vi "RenameVI.vi"(8 "error in (no error)":errorcluster, 11 "InitialName":string) -> (0 "error out":errorcluster, 3 "NewName":string)   [LabVIEW 2018]
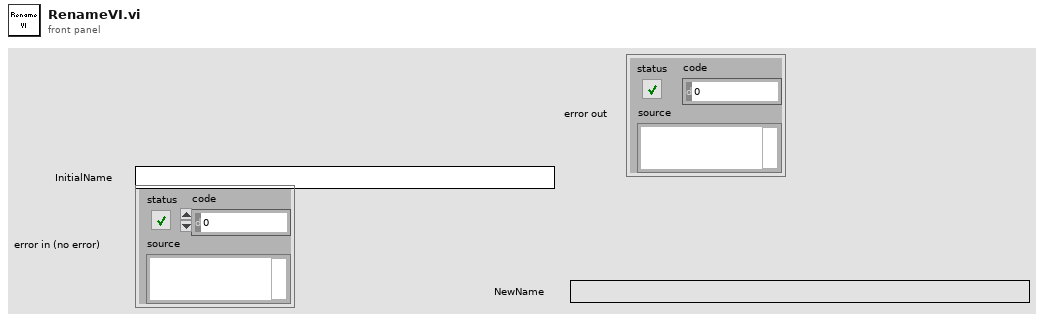
[diagram p1: front panel]
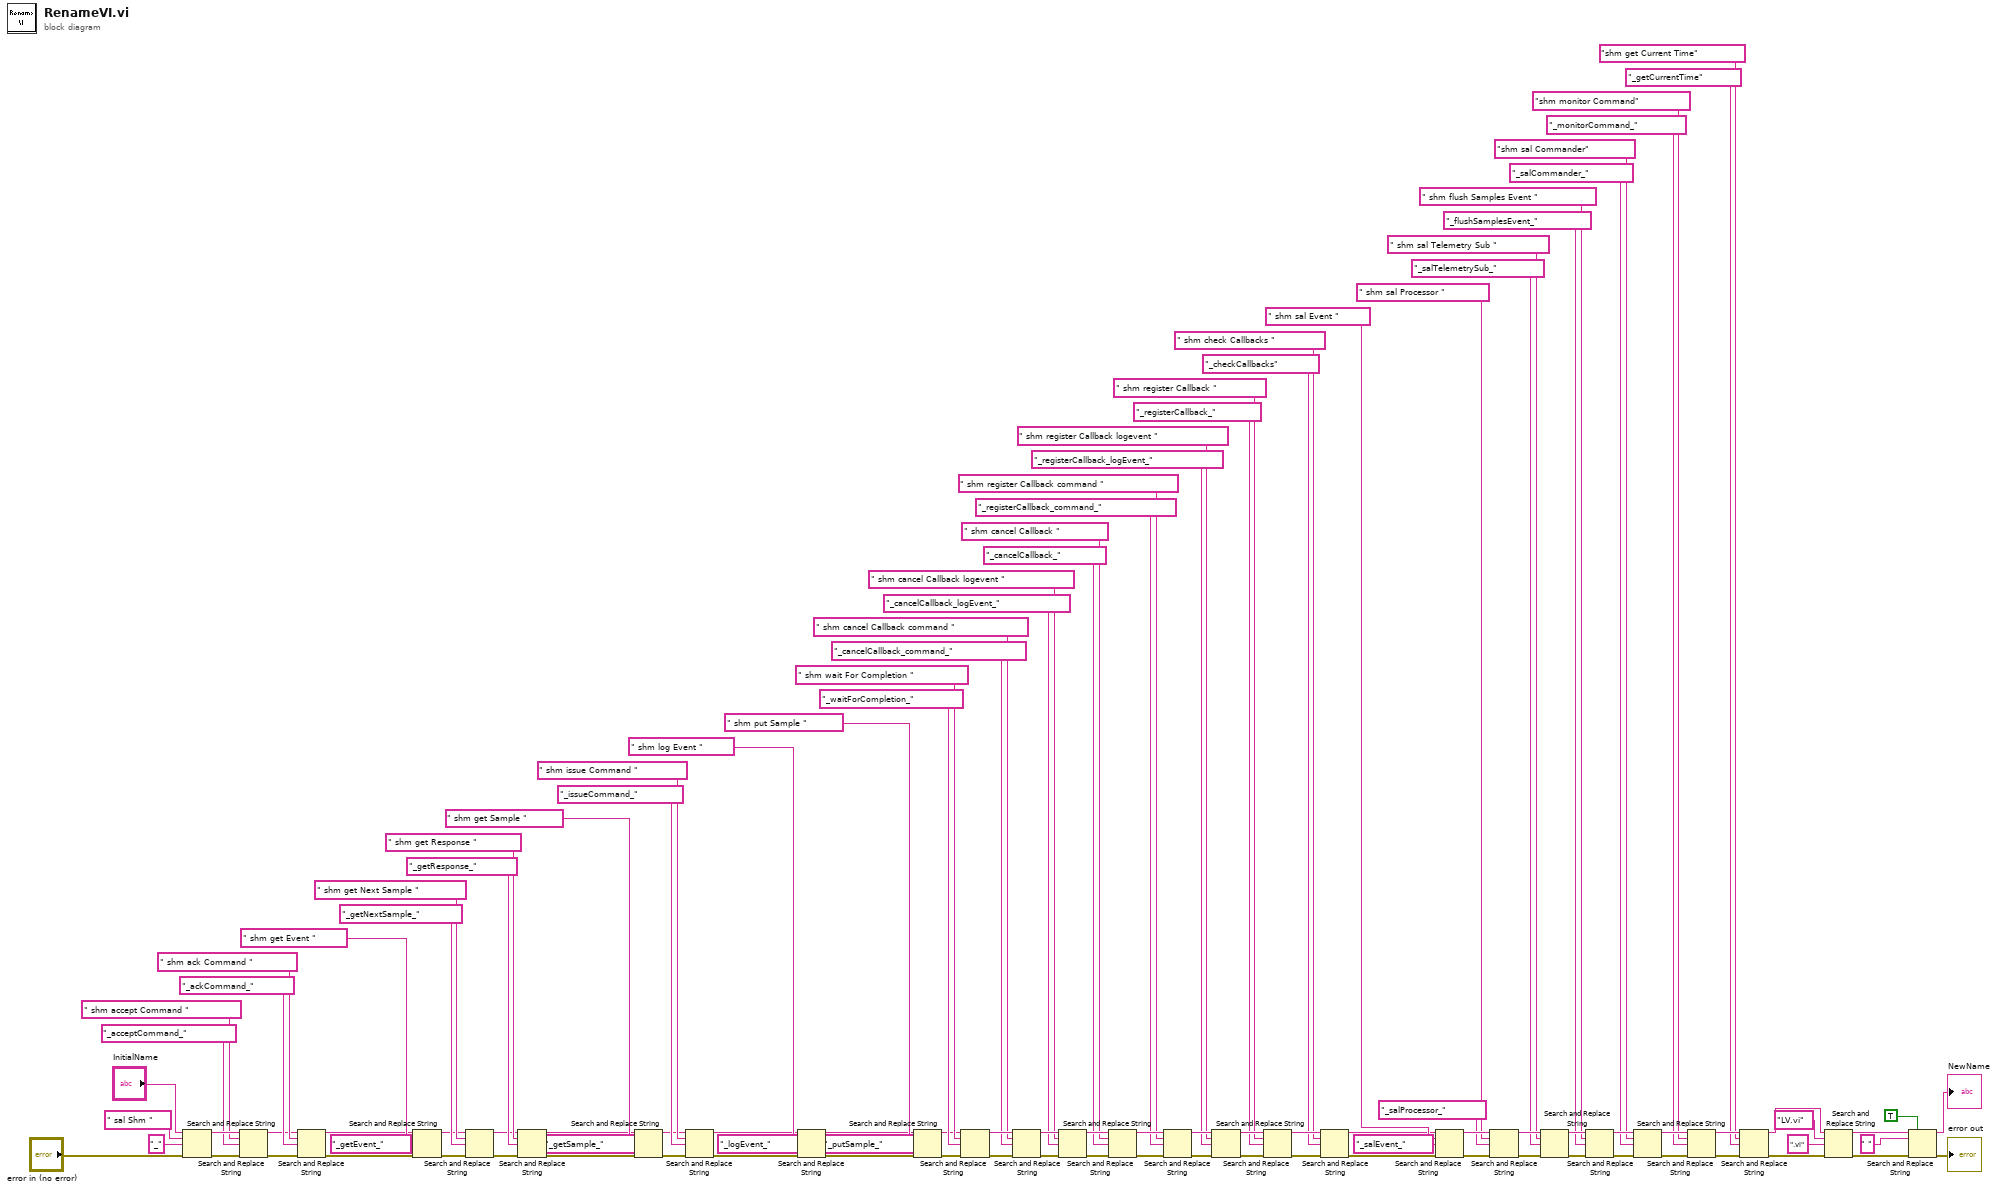
[diagram p0: block diagram]
diagram:
  n1 = Search and Replace String(input string="InitialName", search string=" sal Shm ", replace string="_" ("replace string (\"\")"), error in="error in (no error)") -> (result string=w107:string, error out=w99:errorcluster)  [unwired: 4 in, 2 out]
  n2 = Search and Replace String(input string=w107, search string=" shm accept Command ", replace string="_acceptCommand_" ("replace string (\"\")"), error in=w99) -> (result string=w102:string, error out=w98:errorcluster)  [unwired: 4 in, 2 out]
  n3 = Search and Replace String(input string=w102, search string=" shm ack Command ", replace string="_ackCommand_" ("replace string (\"\")"), error in=w98) -> (result string=w74:string, error out=w97:errorcluster)  [unwired: 4 in, 2 out]
  n4 = Search and Replace String(input string=w74, search string=" shm get Event ", replace string="_getEvent_" ("replace string (\"\")"), error in=w97) -> (result string=w73:string, error out=w94:errorcluster)  [unwired: 4 in, 2 out]
  n5 = Search and Replace String(input string=w73, search string=" shm get Next Sample ", replace string="_getNextSample_" ("replace string (\"\")"), error in=w94) -> (result string=w72:string, error out=w91:errorcluster)  [unwired: 4 in, 2 out]
  n6 = Search and Replace String(input string=w72, search string=" shm get Response ", replace string="_getResponse_" ("replace string (\"\")"), error in=w91) -> (result string=w71:string, error out=w88:errorcluster)  [unwired: 4 in, 2 out]
  n7 = Search and Replace String(input string=w71, search string=" shm get Sample ", replace string="_getSample_" ("replace string (\"\")"), error in=w88) -> (result string=w70:string, error out=w85:errorcluster)  [unwired: 4 in, 2 out]
  n8 = Search and Replace String(input string=w70, search string=" shm issue Command ", replace string="_issueCommand_" ("replace string (\"\")"), error in=w85) -> (result string=w69:string, error out=w82:errorcluster)  [unwired: 4 in, 2 out]
  n9 = Search and Replace String(input string=w69, search string=" shm log Event ", replace string="_logEvent_" ("replace string (\"\")"), error in=w82) -> (result string=w68:string, error out=w79:errorcluster)  [unwired: 4 in, 2 out]
  n10 = Search and Replace String(input string=w68, search string=" shm put Sample ", replace string="_putSample_" ("replace string (\"\")"), error in=w79) -> (result string=w67:string, error out=w76:errorcluster)  [unwired: 4 in, 2 out]
  n11 = Search and Replace String(input string=w67, search string=" shm wait For Completion ", replace string="_waitForCompletion_" ("replace string (\"\")"), error in=w76) -> (result string=w58:string, error out=w57:errorcluster)  [unwired: 4 in, 2 out]
  n12 = Search and Replace String(input string=w58, search string=" shm cancel Callback command ", replace string="_cancelCallback_command_" ("replace string (\"\")"), error in=w57) -> (result string=w54:string, error out=w53:errorcluster)  [unwired: 4 in, 2 out]
  n13 = Search and Replace String(input string=w54, search string=" shm cancel Callback logevent ", replace string="_cancelCallback_logEvent_" ("replace string (\"\")"), error in=w53) -> (result string=w50:string, error out=w49:errorcluster)  [unwired: 4 in, 2 out]
  n14 = Search and Replace String(input string=w50, search string=" shm cancel Callback ", replace string="_cancelCallback_" ("replace string (\"\")"), error in=w49) -> (result string=w46:string, error out=w45:errorcluster)  [unwired: 4 in, 2 out]
  n15 = Search and Replace String(input string=w46, search string=" shm register Callback command ", replace string="_registerCallback_command_" ("replace string (\"\")"), error in=w45) -> (result string=w42:string, error out=w41:errorcluster)  [unwired: 4 in, 2 out]
  n16 = Search and Replace String(input string=w42, search string=" shm register Callback logevent ", replace string="_registerCallback_logEvent_" ("replace string (\"\")"), error in=w41) -> (result string=w38:string, error out=w37:errorcluster)  [unwired: 4 in, 2 out]
  n17 = Search and Replace String(input string=w38, search string=" shm register Callback ", replace string="_registerCallback_" ("replace string (\"\")"), error in=w37) -> (result string=w34:string, error out=w33:errorcluster)  [unwired: 4 in, 2 out]
  n18 = Search and Replace String(input string=w34, search string=" shm check Callbacks ", replace string="_checkCallbacks" ("replace string (\"\")"), error in=w33) -> (result string=w20:string, error out=w19:errorcluster)  [unwired: 4 in, 2 out]
  n19 = Search and Replace String(input string=w20, search string=" shm sal Event ", replace string="_salEvent_" ("replace string (\"\")"), error in=w19) -> (result string=w28:string, error out=w26:errorcluster)  [unwired: 4 in, 2 out]
  n20 = Search and Replace String(input string=w28, search string=" shm sal Processor ", replace string="_salProcessor_" ("replace string (\"\")"), error in=w26) -> (result string=w27:string, error out=w25:errorcluster)  [unwired: 4 in, 2 out]
  n21 = Search and Replace String(input string=w27, search string=" shm sal Telemetry Sub ", replace string="_salTelemetrySub_" ("replace string (\"\")"), error in=w25) -> (result string=w18:string, error out=w17:errorcluster)  [unwired: 4 in, 2 out]
  n22 = Search and Replace String(input string=w18, search string=" shm flush Samples Event ", replace string="_flushSamplesEvent_" ("replace string (\"\")"), error in=w17) -> (result string=w16:string, error out=w15:errorcluster)  [unwired: 4 in, 2 out]
  n23 = Search and Replace String(input string=w16, search string="shm sal Commander", replace string="_salCommander_" ("replace string (\"\")"), error in=w15) -> (result string=w10:string, error out=w9:errorcluster)  [unwired: 4 in, 2 out]
  n24 = Search and Replace String(input string=w10, search string="shm monitor Command", replace string="_monitorCommand_" ("replace string (\"\")"), error in=w9) -> (result string=w3:string, error out=w4:errorcluster)  [unwired: 4 in, 2 out]
  n25 = Search and Replace String(input string=w3, search string="shm get Current Time", replace string="_getCurrentTime" ("replace string (\"\")"), error in=w4) -> (result string=w6:string, error out=w5:errorcluster)  [unwired: 4 in, 2 out]
  n26 = Search and Replace String(input string=w6, search string="LV.vi", replace string=".vi" ("replace string (\"\")"), error in=w5) -> (result string=w64:string, error out=w62:errorcluster)  [unwired: 4 in, 2 out]
  n27 = Search and Replace String(replace all?=TRUE ("replace all? (F)"), input string=w64, search string=" ", error in=w62) -> (result string=→"NewName":string, error out=→"error out":errorcluster)  [unwired: 4 in, 2 out]
